vi "RESTful Boolean To Text.vi"(1 "Boolean":bool) -> (0 "Boolean Text":string)   [LabVIEW 2020]
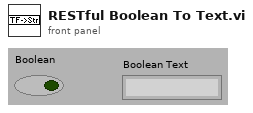
[diagram p1: front panel]
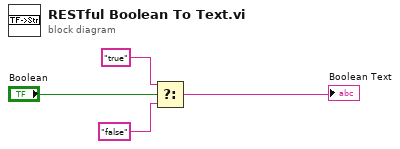
[diagram p0: block diagram]
diagram:
  n1 = Select(t="true", s="Boolean", f="false") -> (s? t:f=→"Boolean Text":string)
